vi "Simple_controller.vi"(0 "Slip ratio from TORCS":dbl, 1 "ordinary brake signal":dbl, 5 "ABS Enable":bool=TRUE, 15 "Front left wheel":dbl(slide)=0.49999999999999994 scale=0.0..1.0, 16 "Rear left wheel":dbl(slide)=0.49999999999999994 scale=0.0..1.0, 17 "Front right wheel":dbl(slide)=0.49999999999999994 scale=0.0..1.0, 19 "Rear right wheel":dbl(slide)=0.49999999999999994 scale=0.0..1.0) -> (14 "Brake signal filtered":dbl, 18 "counter":dbl)   [LabVIEW 2012]
panel:
  out "Brake signal filtered rear right":dbl
  out "Brake signal filtered rear left":dbl
  out "Brake signal filtered front left":dbl
  out "Brake signal filtered front right":dbl
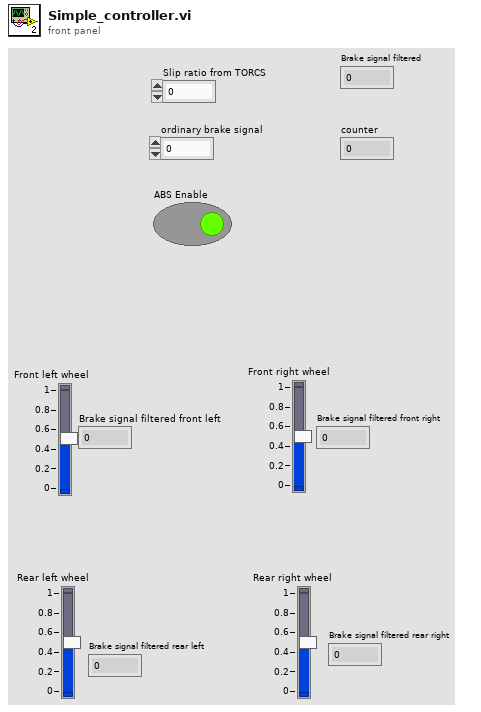
[diagram p1: front panel]
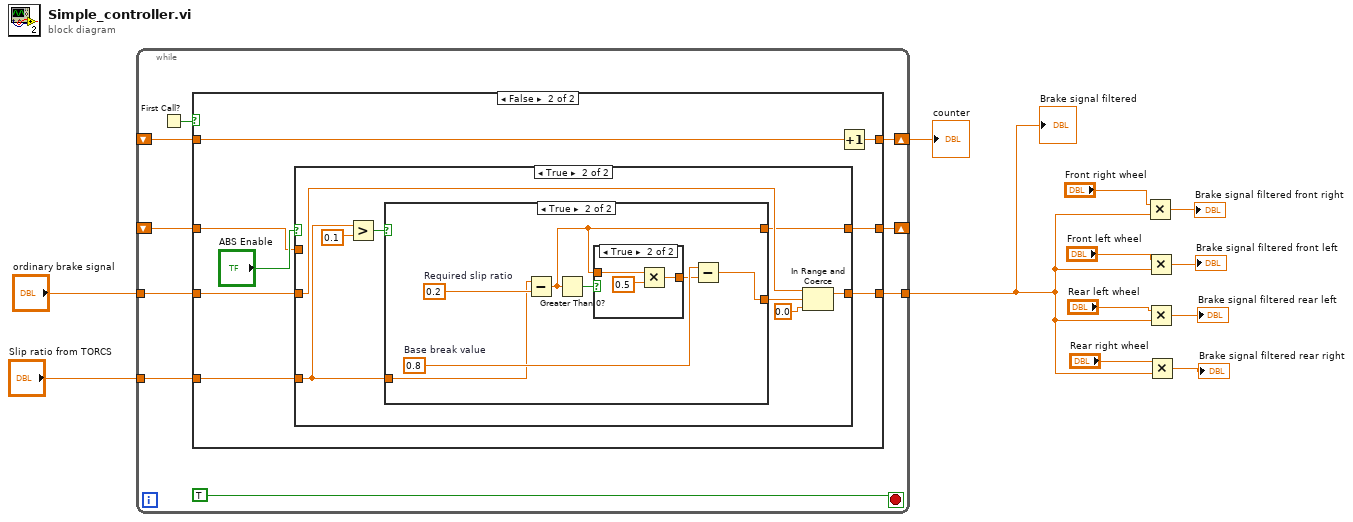
[diagram p0: block diagram]
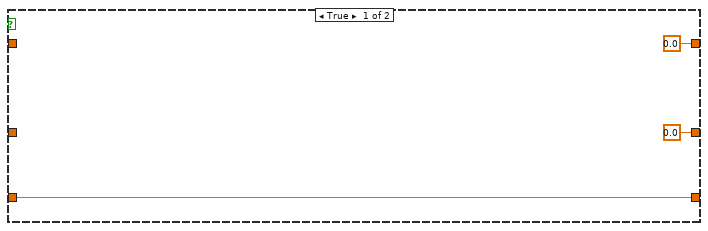
[diagram p2: hidden frame]
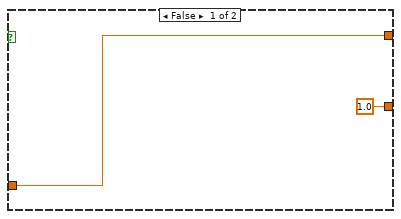
[diagram p4: hidden frame]
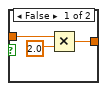
[diagram p5: hidden frame]
diagram:
  n1 = while {
    tunnel: [w20] -> w9
    tunnel: "ordinary brake signal" -> [w19]
    shift-right: [w17] -> w11
    shift-left: _ -> [w16]
    tunnel: "Slip ratio from TORCS" -> [w15]
    shift-right: [w14] -> _
    shift-left: _ -> [w13]
    stop <- TRUE stop-if-true
    n2 = First Call?() -> (First Call?: T/F=w21:bool)
    n3 = case shown="False" w21 {
      tunnel: [w24 w29] -> w20
      tunnel: w19 -> [w24 w28]
      tunnel: [0.0 ("counter") w30] -> w17
      tunnel: w16 -> [_ w31]
      tunnel: w15 -> [_ w27]
      tunnel: [0.0 ("counter") w26] -> w14
      tunnel: w13 -> [_ w25]
      frame True {
      }
      frame False {
        n4 = case shown="True" "ABS Enable" {
          tunnel: [w34 w42] -> w29
          tunnel: w28 -> [w34 w41]
          tunnel: w27 -> [_ w38]
          tunnel: [w33 w40] -> w26
          tunnel: w25 -> [w33 _]
          frame False {
          }
          frame True {
            n5 = Greater?(x=w38, y=0.1) -> (0:w35:bool)
            n6 = case shown="True" w35 {
              tunnel: [w43 w47] -> w40
              tunnel: [1.0 w45] -> w39
              tunnel: w38 -> [w43 w46]
              frame False {
              }
              frame True {
                w50 = 0.8  # Base break value
                w51 = 0.2  # Required slip ratio
                n7 = Subtract(x=w46, y=w51) -> (x-y=w47:dbl)
                n8 = Greater Than 0?(x=w47) -> (x > 0?=w48:bool)
                n9 = case shown="True" w48 {
                  tunnel: w47 -> [w53 w57]
                  tunnel: [w52 w55] -> w49
                  frame False {
                    n10 = Multiply(x=w53, y=2.0) -> (x*y=w52:dbl)
                  }
                  frame True {
                    n11 = Multiply(x=w57, y=0.5) -> (x*y=w55:dbl)
                  }
                }
                n12 = Subtract(x=w50, y=w49) -> (x-y=w45:dbl)
              }
            }
            n13 = In Range and Coerce(upper limit=w41, x=w39, lower limit=0.0) -> (coerced(x)=w42:dbl)  [unwired: 1 out]
          }
        }
        n14 = Increment(x=w31) -> (x+1=w30:dbl)
      }
    }
  }
  "Brake signal filtered" <- w9
  "counter" <- w11
  n15 = Multiply(x="Front right wheel", y=w9) -> (x*y=→"Brake signal filtered front right":dbl)
  n16 = Multiply(x="Front left wheel", y=w9) -> (x*y=→"Brake signal filtered front left":dbl)
  n17 = Multiply(x="Rear left wheel", y=w9) -> (x*y=→"Brake signal filtered rear left":dbl)
  n18 = Multiply(x="Rear right wheel", y=w9) -> (x*y=→"Brake signal filtered rear right":dbl)
